vi "Launch UI.vi"(8 "error in (no error)":errorcluster, 11 "Controller In":refnum<class "Controller.lvclass">) -> (0 "error out":errorcluster, 3 "Controller Out":refnum<class "Controller.lvclass">)   [LabVIEW 2017, in "Controller Actor.lvlib" / "Controller.lvclass"]
uses:
  Controller.lvclass
  C:/Program Files (x86)/National Instruments/LabVIEW 2017/vi.lib/ActorFramework/Actor/Actor.lvclass
  User Interface/UI.lvclass
  <vilib>/ActorFramework/Actor/Actor.lvclass
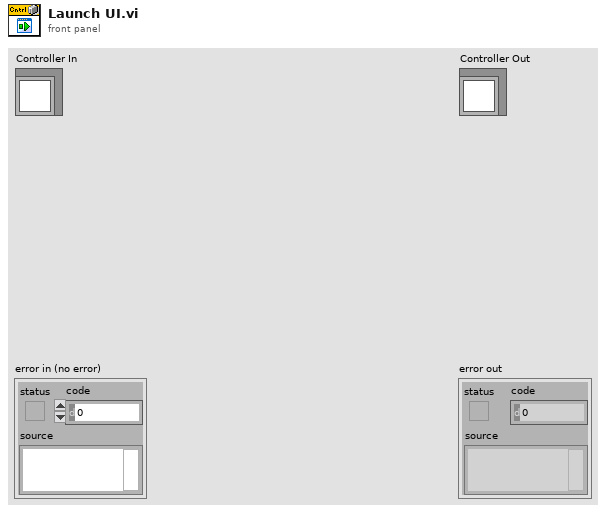
[diagram p1: front panel]
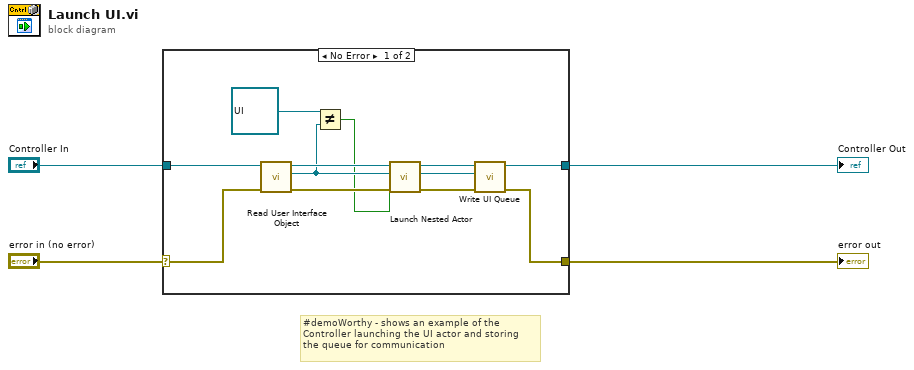
[diagram p0: block diagram]
diagram:
  # "#demoWorthy - shows an example of the \nController launching the UI actor and storing\nthe queue for communication"
  n1 = case shown="No Error" "error in (no error)" {
    selector: "error in (no error)" -> [w14 w18]
    tunnel: [w13 w18] -> w3
    tunnel: [w16 w17] -> w1
    tunnel: "Controller In" -> [w15 w17]
    frame No Error {
      n2 = call "Read User Interface Object.vi"("error in (no error)"=w14, "UI Controller in"=w15) -> ("error out"=w10:errorcluster, "UI.lvclass"=w7:refnum<class "UI.lvclass">, "UI Controller out"=w8:refnum<class "Controller.lvclass">)  [unwired: 7 in]
      n3 = Not Equal?(x=refnum<class "UI.lvclass"> refnum ("Generic UI Actor.lvlib:UI.lvclass"), y=w7) -> (x != y?=w6:bool)
      n4 = call <vilib>:"Launch Nested Actor.vi"("Open Actor Core front panel? (F)"=w6, "error in (no error)"=w10, "Nested Actor"=w7, "Caller Actor in"=w8) -> ("error out"=w11:errorcluster, "Nested Actor's Enqueuer"=w12:refnum<class "Message Enqueuer.lvclass">, "Caller Actor out"=w9:refnum<class "Controller.lvclass">)  [unwired: 5 in]
      n5 = call "Write UI Queue.vi"("error in (no error)"=w11, "UI Queue"=w12, "UI Controller in"=w9) -> ("error out"=w13:errorcluster, "UI Controller out"=w16:refnum<class "Controller.lvclass">)  [unwired: 7 in]
    }
    frame Error {
    }
  }
  "error out" <- w3
  "Controller Out" <- w1
